vi "TCP HTTP test.vi"() -> ()   [LabVIEW 2015]
panel:
  out "body":string
  out "header":string
  out "error out":errorcluster
  in  "URL":string="http://localhost:24414"
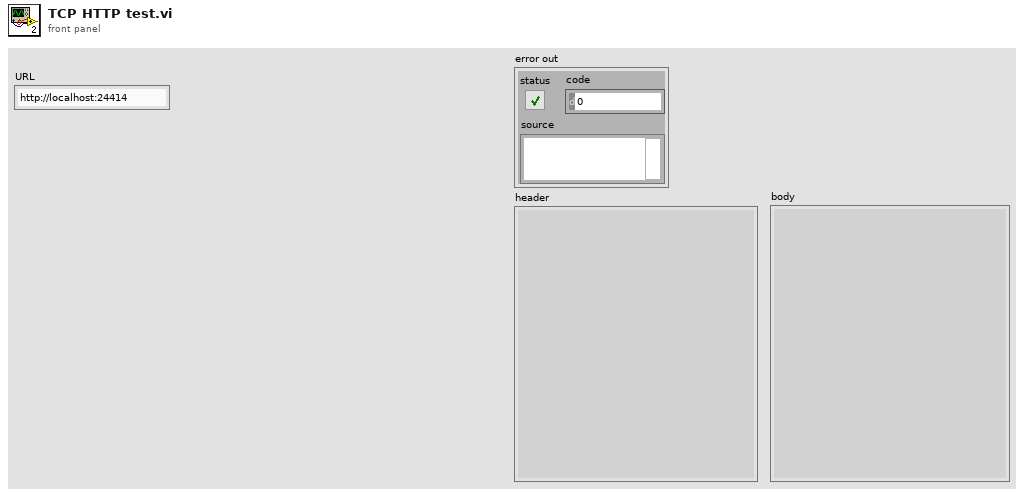
[diagram p1: front panel]
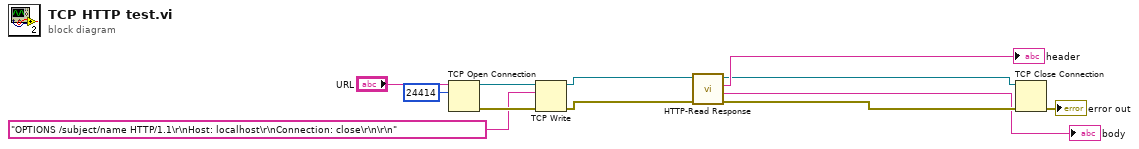
[diagram p0: block diagram]
diagram:
  n1 = TCP Open Connection(address="URL", remote port or service name=u16 24414) -> (connection ID=w9:refnum<k5>, error out=w8:errorcluster)  [unwired: 3 in]
  n2 = TCP Write(connection ID=w9, data in="OPTIONS /subject/name HTTP/1.1\r\nHost: localhost\r\nConnection: close\r\n\r\n", error in (no error)=w8) -> (connection ID out=w6:refnum<k5>, error out=w7:errorcluster)  [unwired: 1 in, 1 out]
  n3 = call "HTTP-Read Response.vi"("error in (no error)"=w7, "TCP Network Connection in"=w6) -> ("error out"=w2:errorcluster, "Body"=→"body":string, "Header"=→"header":string, "TCP Network Connection out"=w3:refnum<k5>)  [unwired: 6 in]
  n4 = TCP Close Connection(connection ID=w3, error in (no error)=w2) -> (error out=→"error out":errorcluster)  [unwired: 1 in, 1 out]
